vi "Write Uml.vi"(8 "error in (no error)":errorcluster, 10 "Uml":string, 11 "object in":refnum<class "TAFConfiguration.lvclass">) -> (0 "error out":errorcluster, 3 "object out":refnum<class "TAFConfiguration.lvclass">)   [LabVIEW 2021, in "TAF Proj Document Type.lvlib" / "TAFConfiguration.lvclass"]
uses:
  <vilib>/Wovalab/AntiDoc/Document Type/Add-ons/LabVIEW TAF Project/TAFConfiguration/TAFConfiguration.lvclass
  <vilib>/Wovalab/AntiDoc/Document Type/Add-ons/LabVIEW TAF Project/TAFConfiguration/TAFConfiguration.lvclass/TAFConfiguration.ctl
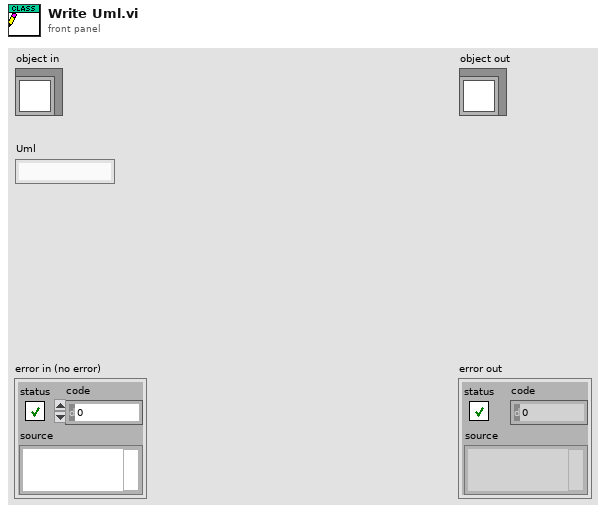
[diagram p1: front panel]
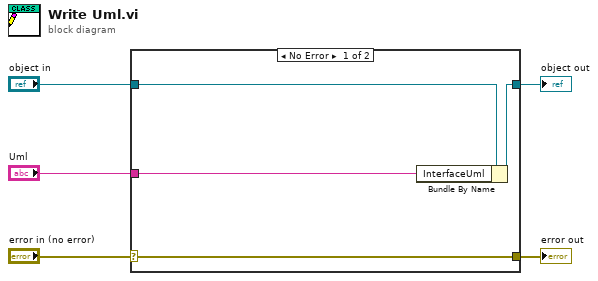
[diagram p0: block diagram]
diagram:
  n1 = case shown="No Error" "error in (no error)" {
    selector: "error in (no error)" -> [w9 w10]
    tunnel: [w9 w10] -> w4
    tunnel: [w7 w11] -> w2
    tunnel: "object in" -> [w8 w11]
    tunnel: "Uml" -> [w6 _]
    frame No Error {
      n2 = Bundle By Name(cluster=w8, "InterfaceUml"=w6) -> (w7:refnum<class "TAFConfiguration.lvclass">)
    }
    frame Error {
    }
  }
  "error out" <- w4
  "object out" <- w2
